vi "change_image_position.vi"(10 "position":cluster{"left":i32, "top":i32}, 11 "image data in":T1) -> (3 "image data out":T1)   [LabVIEW 2025]
uses:
  <vilib>/picture/picture.llb/imagedata.ctl
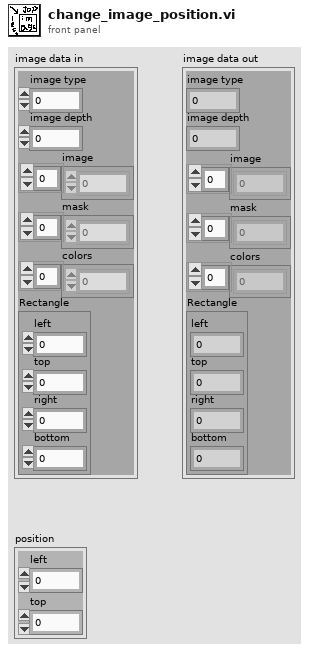
[diagram p1: front panel]
types:
  T1 = typedef "imagedata.ctl" = cluster{"image type":i32, "image depth":i32, "image":u8[], "mask":u8[], "colors":u32[], "Rectangle":cluster{"left":i16, "top":i16, "right":i16, "bottom":i16}}
  T2 = cluster{"left":i16, "top":i16, "right":i16, "bottom":i16}
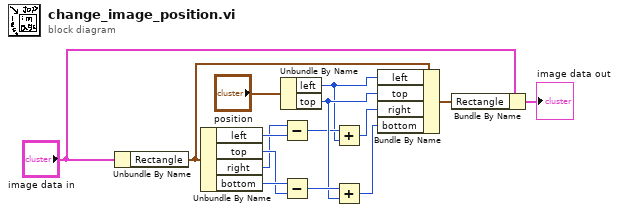
[diagram p0: block diagram]
diagram:
  n1 = Unbundle By Name("image data in") -> ("Rectangle"=w2:T2)
  n2 = Unbundle By Name(w2) -> ("left"=w6:i16, "top"=w11:i16, "right"=w5:i16, "bottom"=w12:i16)
  n3 = Unbundle By Name("position") -> ("left"=w3:i32, "top"=w9:i32)
  n4 = Subtract(x=w5, y=w6) -> (x-y=w4:i16)
  n5 = Subtract(x=w12, y=w11) -> (x-y=w10:i16)
  n6 = Add(x=w4, y=w3) -> (x+y=w7:i32)
  n7 = Add(x=w10, y=w9) -> (x+y=w8:i32)
  n8 = Bundle By Name(cluster=w2, "left"=w3, "top"=w9, "right"=w7, "bottom"=w8) -> (w15:T2)
  n9 = Bundle By Name(cluster="image data in", "Rectangle"=w15) -> (→"image data out":T1)
